vi "Get RT INI.vi"(8 "error in (no error)":errorcluster, 10 "Non-default local path":path, 11 "RT Management in":refnum<class "RT Management.lvclass">) -> (0 "error out":errorcluster, 2 "Local RT INI path":path, 3 "RT Management out":refnum<class "RT Management.lvclass">)   [LabVIEW 2015, in "RT Management.lvlib" / "RT Management.lvclass"]
doc: "Gets the RT INI and places it at a local path. The default location for PharLap and VxWorks targets is \"ni-rt.ini\" and for Linux targets is \"etc/natinst/share/ni-rt.ini\".\n\nThe Non-default local path control is only intended to be used if the user wants to keep the local file."
uses:
  RT Management.lvclass
  RT Management.lvclass/RT Management.ctl
  Get SysCfg Session.vi
  File Transfer Behavior/File Transfer Behavior.lvclass
  <resource>/objmgr/nisysapi.rc
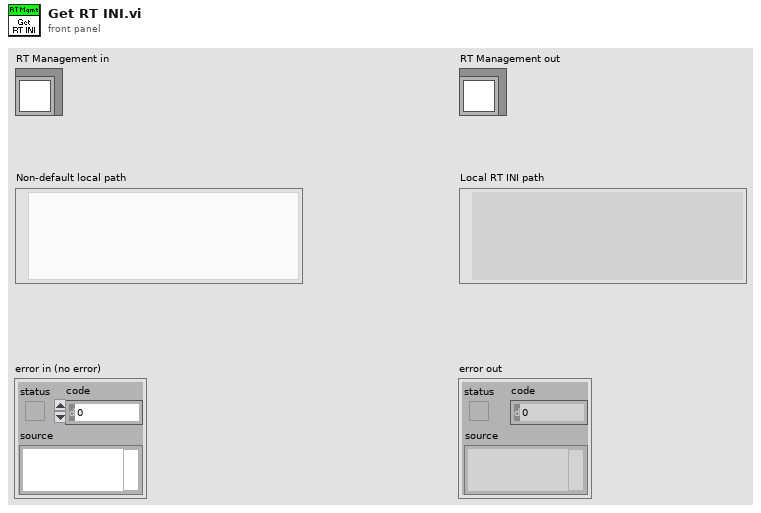
[diagram p1: front panel]
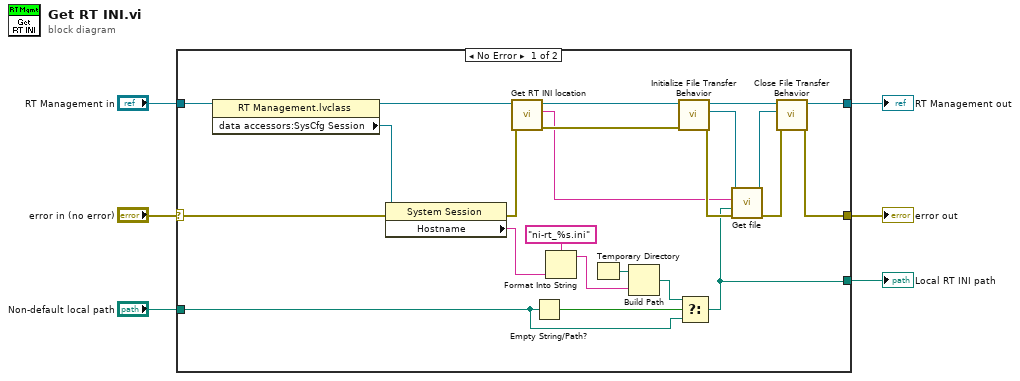
[diagram p0: block diagram]
diagram:
  n1 = case shown="No Error" "error in (no error)" {
    selector: "error in (no error)" -> [w17 w31]
    tunnel: [w7 w31] -> w5
    tunnel: [w15 w30] -> w3
    tunnel: "RT Management in" -> [w18 w30]
    tunnel: [w19 _] -> w2
    tunnel: "Non-default local path" -> [w20 _]
    frame No Error {
      n2 = property class="RT Management.lvclass"(reference=w18) -> (reference out=w12:refnum<class "RT Management.lvclass">, "data accessors:SysCfg Session"=w24:refnum<k21>)  [unwired: 1 in, 1 out]
      n3 = property class="System Session"(reference=w24, error in=w17) -> (error out=w9:errorcluster, "Hostname"=w26:string)  [unwired: 1 out]
      n4 = call "Get RT INI location.vi"("error in (no error)"=w9, "RT Management in"=w12) -> ("error out"=w29:errorcluster, "RT INI Location"=w10:string, "RT Management out"=w11:refnum<class "RT Management.lvclass">)  [unwired: 7 in]
      n5 = Empty String/Path?(string/path=w20) -> (empty?=w21:bool)
      n6 = Format Into String(format string="ni-rt_%s.ini" ("name or relative path"), w26) -> (resulting string=w25:string)  [unwired: 2 in, 1 out]
      n7 = Temporary Directory() -> (w23:path)
      n8 = Build Path(base path=w23, name or relative path=w25) -> (appended path=w22:path)
      n9 = call "Initialize File Transfer Behavior.vi"("error in (no error)"=w29, "RT Management in"=w11) -> ("error out"=w28:errorcluster, "File Transfer Behavior out"=w14:refnum<class "File Transfer Behavior.lvclass">, "RT Management out"=w13:refnum<class "RT Management.lvclass">)  [unwired: 7 in]
      n10 = Select(t=w22, s=w21, f=w20) -> (s? t:f=w19:path)
      n11 = call-dynamic "Get file.vi"("error in (no error)"=w28, "Local path"=w19, "Remote path"=w10, "File Transfer Behavior in"=w14) -> ("error out"=w8:errorcluster, "File Transfer Behavior out"=w16:refnum<class "File Transfer Behavior.lvclass">)  [unwired: 6 in]
      n12 = call "Close File Transfer Behavior.vi"("error in (no error)"=w8, "File Transfer Behavior in"=w16, "RT Management in"=w13) -> ("error out"=w7:errorcluster, "RT Management out"=w15:refnum<class "RT Management.lvclass">)  [unwired: 7 in]
    }
    frame Error {
    }
  }
  "error out" <- w5
  "RT Management out" <- w3
  "Local RT INI path" <- w2
